vi "Norm VI Pt 2.vi"() -> ()   [LabVIEW 2026]
uses:
  <vilib>/DAQmx/read.llb/DAQmx Read (Digital 1D Bool 1Chan 1Samp).vi
  <vilib>/DAQmx/write.llb/DAQmx Write (Digital 1D Bool 1Chan 1Samp).vi
  <vilib>/numeric/Random Number (Range) U64.vi
  <vilib>/numeric/sub_Random U32.vi
  <vilib>/DAQmx/create/channels.llb/DAQmx Create Channel (DO-Digital Output).vi
  <vilib>/DAQmx/create/channels.llb/DAQmx Create Channel (DI-Digital Input).vi
  <vilib>/DAQmx/miscellaneous.llb/DAQmx Fill In Error Info.vi
panel:
  in  "stop":bool
  out "error out 5":errorcluster
  out "Numeric":i32
  out "Player 2":u64
  out "error out 4":errorcluster
  out "error out 3":errorcluster
  out "First Press?  2":bool
  out "Previous LED Position 2":u64
  out "Iteration Count 2":i32
  out "LEDs 2":bool[](array[boolean])
  out "HW Buttons  2":bool[](array[boolean])
  in  "?":bool
  in  "SW Buttons 2":bool[](array[boolean])
  out "Player 1":i8
  out "error out 2":errorcluster
  out "error out":errorcluster
  in  "SW Buttons":bool[](array[boolean])
  out "Debug Mode?":bool=TRUE
  out "First Press?":bool
  out "Previous LED Position":u64
  in  "Stop Program":bool
  out "HW Buttons":bool[](array[boolean])
  out "Iteration Count":i32
  out "LEDs":bool[](array[boolean])
  # "NI Speed of Light Demo"
  # "Press (Sticky Note) Button to Begin!"
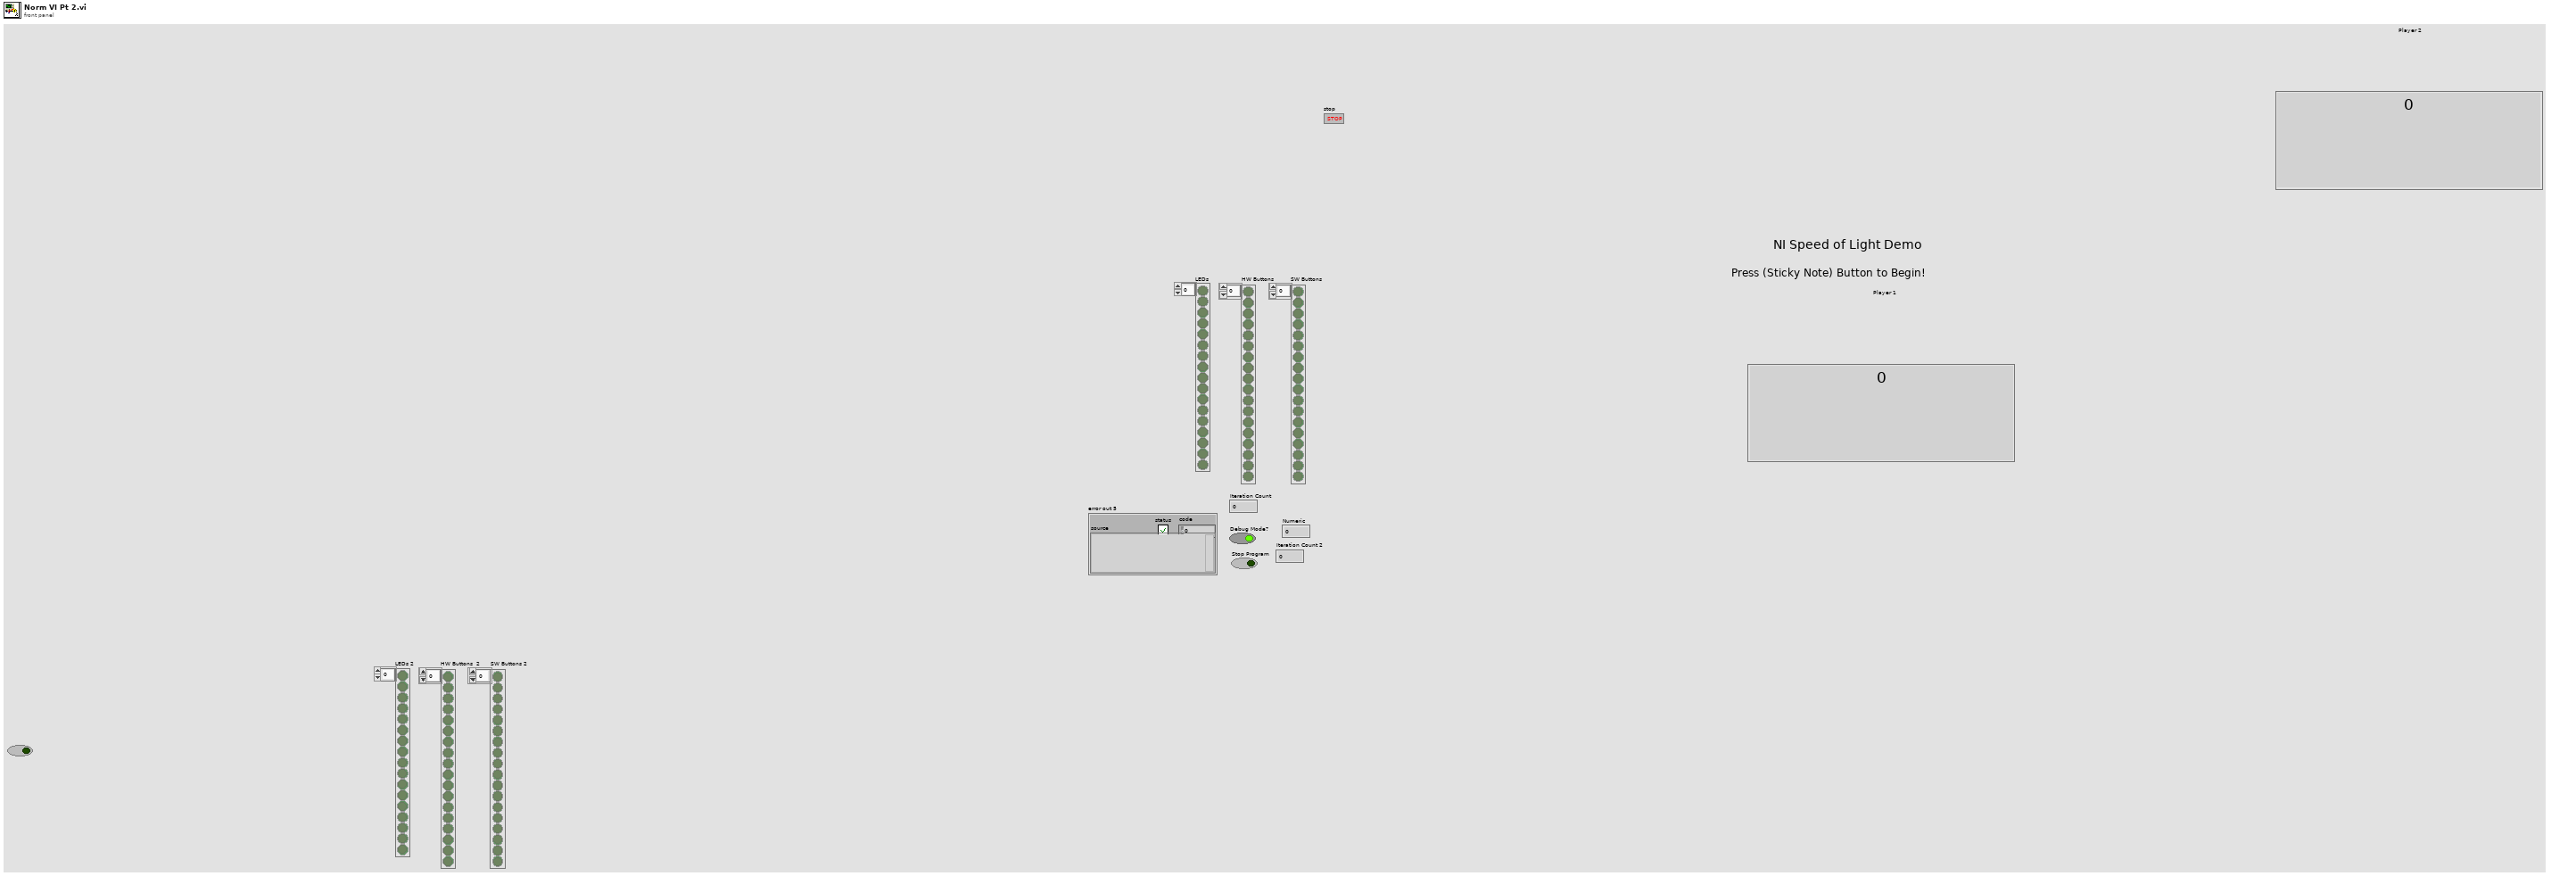
[diagram p1: front panel]
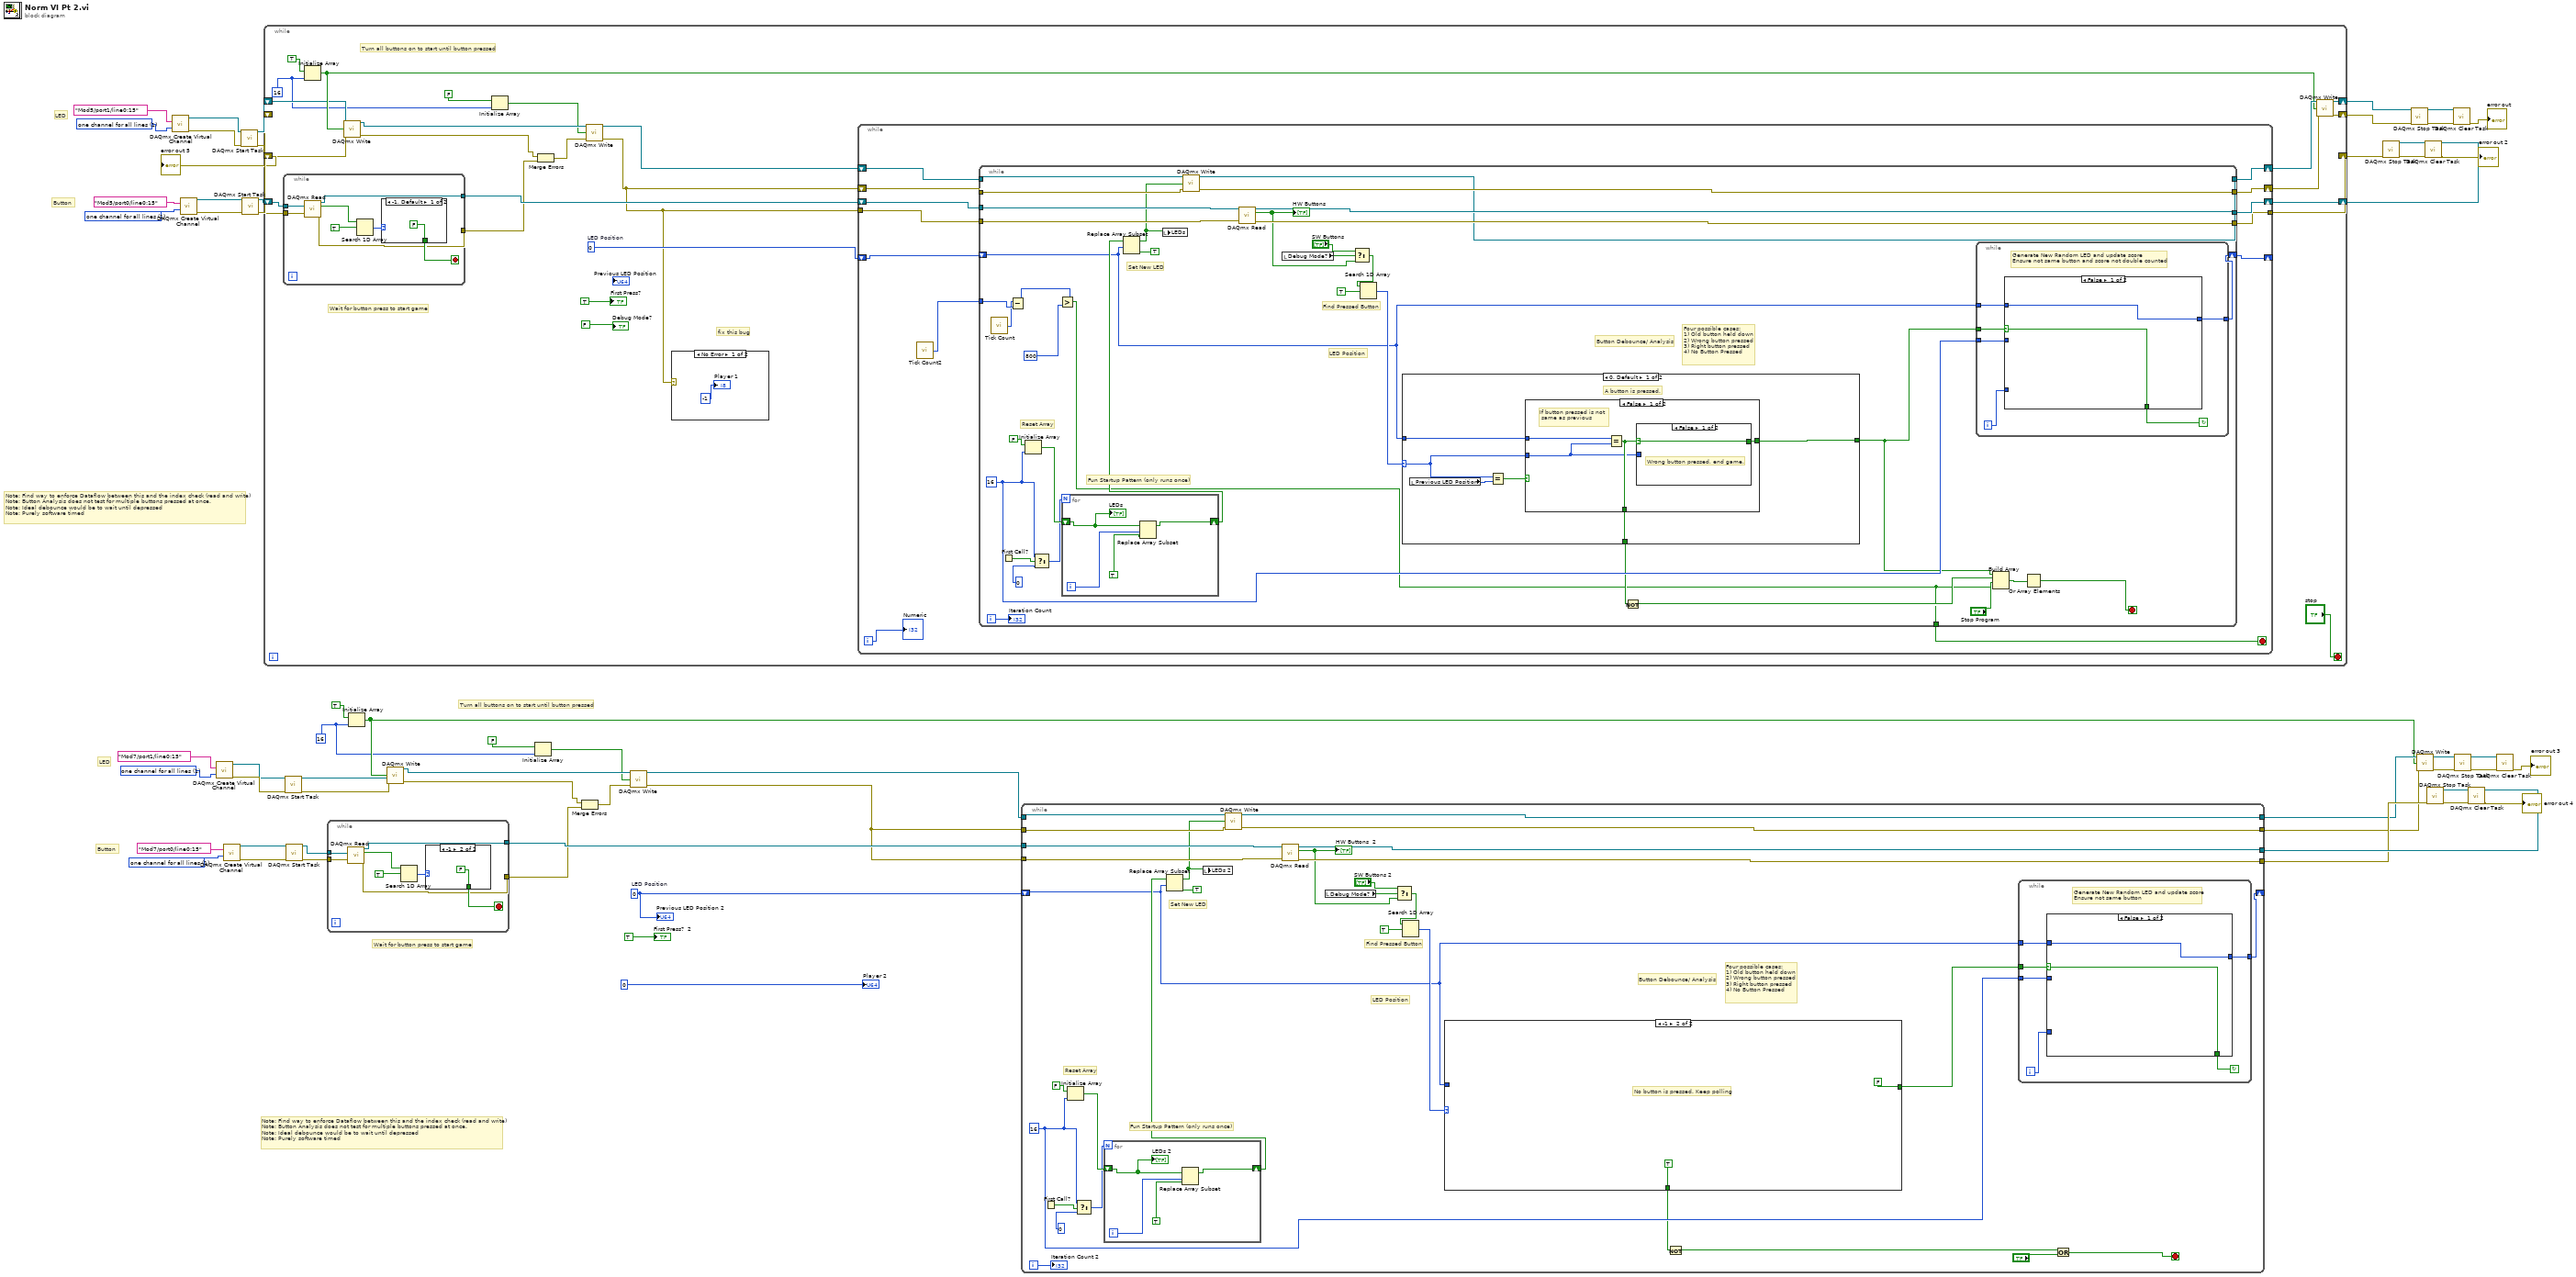
[diagram p0: block diagram]
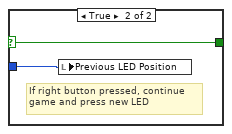
[diagram p3: hidden frame]
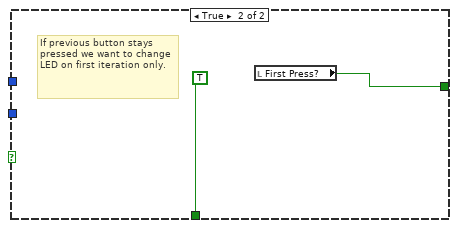
[diagram p4: hidden frame]
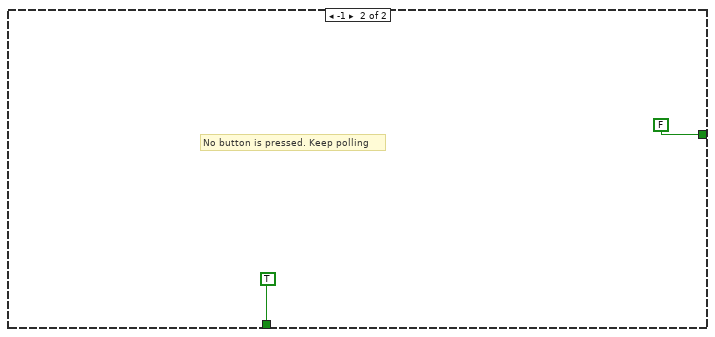
[diagram p5: hidden frame]
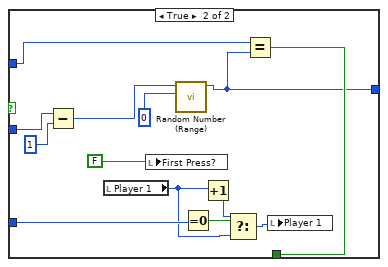
[diagram p6: hidden frame]
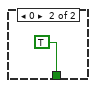
[diagram p7: hidden frame]
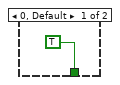
[diagram p8: hidden frame]
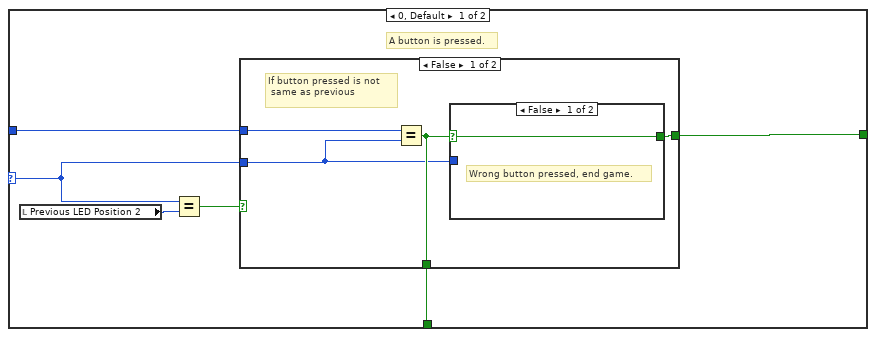
[diagram p9: hidden frame]
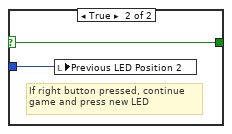
[diagram p10: hidden frame]
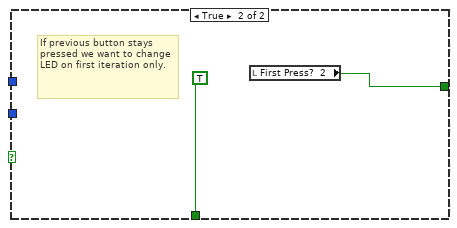
[diagram p11: hidden frame]
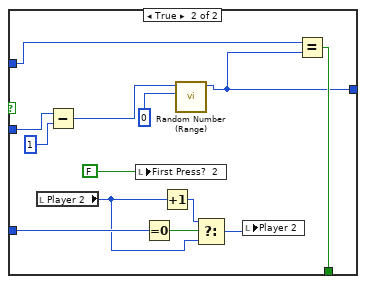
[diagram p12: hidden frame]
diagram:
  w6 = 16 ("dimension size")
  w28 = 1 items=["one channel for each line", "one channel for all lines"] ("line grouping")
  w29 = 1 items=["one channel for each line", "one channel for all lines"] ("line grouping")
  w27 = u64 0  # LED Position
  w50 = 1 items=["one channel for each line", "one channel for all lines"] ("line grouping")
  w51 = 1 items=["one channel for each line", "one channel for all lines"] ("line grouping")
  # "Turn all buttons on to start until button pressed"
  # "Wait for button press to start game"
  # "Note: Find way to enforce Dataflow between this and the index check (read and write)\nNote: Button Analysis does not test for multiple buttons pressed at once. \nNote: Ideal debounce would be to wait until depressed\nNote: Purely software timed"
  # "LED"
  # "Button"
  # "Note: Find way to enforce Dataflow between this and the index check (read and write)\nNote: Button Analysis does not test for multiple buttons pressed at once. \nNote: Ideal debounce would be to wait until depressed\nNote: Purely software timed"
  # "LED"
  # "Button"
  n1 = call-poly <vilib>:"DAQmx Create Virtual Channel.vi"("lines"=tag "Mod5/port1/line0:15", "line grouping"=w51) -> ("task out"=w3:refnum<k21>, "error out"=w2:errorcluster)  [unwired: 12 in]
  n2 = call-poly <vilib>:"DAQmx Create Virtual Channel.vi"("lines"=tag "Mod5/port0/line0:15", "line grouping"=w50) -> ("task out"=w60:refnum<k21>, "error out"=w61:errorcluster)  [unwired: 12 in]
  n3 = call-poly <vilib>:"DAQmx Create Virtual Channel.vi"("lines"=tag "Mod7/port1/line0:15", "line grouping"=w29) -> ("task out"=w35:refnum<k21>, "error out"=w36:errorcluster)  [unwired: 12 in]
  n4 = call-poly <vilib>:"DAQmx Create Virtual Channel.vi"("lines"=tag "Mod7/port0/line0:15", "line grouping"=w28) -> ("task out"=w41:refnum<k21>, "error out"=w42:errorcluster)  [unwired: 12 in]
  n5 = call <vilib>:"DAQmx Start Task.vi"("task/channels in"=w3, "error in"=w2) -> ("task out"=w45:refnum<k21>, "error out"=w1:errorcluster)  [unwired: 12 in]
  "error out 5" <- w1
  n6 = call <vilib>:"DAQmx Start Task.vi"("task/channels in"=w60, "error in"=w61) -> ("task out"=w43:refnum<k21>, "error out"=w44:errorcluster)  [unwired: 12 in]
  n7 = while {
    shift-right: [w82] -> w49
    shift-left: w45 -> [w77]
    shift-right: [w80] -> w48
    shift-left: w44 -> [w76]
    shift-right: [w87] -> w59
    shift-left: w43 -> [w75]
    shift-right: [w86] -> w56
    shift-left: w1 -> [w65]
    stop <- "stop" stop-if-true
    w68 = 16 ("dimension size")
    w64 = u64 0  # LED Position
    # "fix this bug"
    # "Turn all buttons on to start until button pressed"
    # "Wait for button press to start game"
    n8 = while {
      tunnel: w76 -> [w188]
      tunnel: w75 -> [w187]
      tunnel: [w182] -> w72
      tunnel: [w181] -> w74
      stop <- w183 stop-if-true
      n9 = call-poly <vilib>:"DAQmx Read.vi"("task/channels in"=w187, "error in"=w188) -> ("task out"=w181:refnum<k21>, "data"=w186:bool[], "error out"=w182:errorcluster)  [unwired: 11 in]
      n10 = Search 1D Array(1D array=w186, element=TRUE) -> (index of element=w184:i32)  [unwired: 1 in]
      n11 = case shown="-1, Default" w184 {
        tunnel: [FALSE TRUE] -> w183
        frame -1, Default {
        }
        frame 0 {
        }
      }
    }
    n12 = Initialize Array(TRUE, w68) -> (w78:bool[])
    n13 = call-poly <vilib>:"DAQmx Write.vi"("task/channels in"=w77, "data"=w78, "error in"=w65) -> ("task out"=w70:refnum<k21>, "error out"=w73:errorcluster)  [unwired: 10 in, 1 out]
    n14 = Initialize Array(FALSE ("element"), w68) -> (w66:bool[])
    n15 = Merge Errors(w73, w72) -> (w71:errorcluster)
    n16 = call-poly <vilib>:"DAQmx Write.vi"("task/channels in"=w70, "data"=w66, "error in"=w71) -> ("task out"=w69:refnum<k21>, "error out"=w62:errorcluster)  [unwired: 10 in, 1 out]
    n17 = case shown="No Error" w62 {
      frame No Error {
        "Player 1" <- i8 -1 ("Player 3")
      }
      frame Error {
      }
    }
    n18 = while {
      tunnel: [w100] -> w86
      shift-right: [w101] -> w87
      shift-left: w74 -> [w97]
      shift-right: [w98] -> w81
      shift-left: w62 -> [w96]
      shift-right: [w99] -> w85
      shift-left: w69 -> [w95]
      tunnel: w62 -> [w94]
      shift-right: [w91] -> _
      shift-left: w64 -> [w90]
      i -> [w93]
      stop <- w89 stop-if-true
      n19 = call "Tick Count2"() -> ("Tick Count(mSec)"=w92:u32)
      n20 = while {
        shift-right: [w136] -> w91
        shift-left: w90 -> [w118]
        tunnel: w94 -> [w135]
        tunnel: w97 -> [w134]
        tunnel: [w133] -> w101
        tunnel: [w132] -> w100
        tunnel: w96 -> [w131]
        tunnel: w95 -> [w130]
        tunnel: [w129] -> w98
        tunnel: [w128] -> w99
        tunnel: w92 -> [w104]
        tunnel: [w102] -> w89
        i -> [w138]
        stop <- w107 stop-if-true
        w122 = u64 16
        # "LED Position"
        # "Find Pressed Button"
        # "Four possible cases:\n1) Old button held down\n2) Wrong button pressed\n3) Right button pressed\n4) No Button Pressed"
        # "Fun Startup Pattern (only runs once)"
        # "Button Debounce/ Analysis"
        # "Set New LED"
        # "Reset Array"
        n21 = call "Tick Count"() -> ("Tick Count(mSec)"=w103:u32)
        n22 = First Call?() -> (First Call?: T/F=w125:bool)
        n23 = Subtract(x=w103, y=w104) -> (x-y=w106:u32)
        n24 = Initialize Array(FALSE, w122) -> (w126:bool[])
        n25 = Select(t=w122, s=w125, f=u64 0) -> (s? t:f=w123:u64)
        n26 = Greater?(x=w106, y=800) -> (0:w102:bool)
        n27 = for {
          N: w123 -> [_]
          shift-right: [w159] -> w121
          shift-left: w126 -> [w156]
          i -> [w158]
          n28 = Replace Array Subset(array=w156, new element=TRUE ("new element/subarray"), index=w158) -> (w159:bool[])
          "LEDs" <- w156
        }
        n29 = Replace Array Subset(array=w121, new element=TRUE ("new element/subarray"), index=w118) -> (w112:bool[])
        n30 = local write "LEDs"(w112) -> ()
        n31 = call-poly <vilib>:"DAQmx Write.vi"("task/channels in"=w130, "data"=w112, "error in"=w131) -> ("task out"=w128:refnum<k21>, "error out"=w129:errorcluster)  [unwired: 10 in, 1 out]
        n32 = call-poly <vilib>:"DAQmx Read.vi"("task/channels in"=w134, "error in"=w135) -> ("task out"=w133:refnum<k21>, "data"=w114:bool[], "error out"=w132:errorcluster)  [unwired: 11 in]
        "HW Buttons" <- w114
        n33 = local read "Debug Mode?"() -> (w116:bool)
        n34 = Select(t="SW Buttons", s=w116, f=w114) -> (s? t:f=w113:bool[])
        n35 = Search 1D Array(1D array=w113, element=TRUE) -> (index of element=w119:i32)  [unwired: 1 in]
        n36 = case shown="0, Default" w119 {
          selector: w119 -> [w140 _]
          tunnel: [w143 FALSE] -> w109
          tunnel: w118 -> [w141 _]
          tunnel: [w142 TRUE] -> w117
          frame 0, Default {
            # "A button is pressed."
            n37 = local read "Previous LED Position"() -> (w139:u64)
            n38 = Equal?(x=w140, y=w139) -> (x = y?=w144:bool)
            n39 = case shown="False" w144 {
              tunnel: [w145 w152] -> w143
              tunnel: [w147 TRUE] -> w142
              tunnel: w140 -> [w146 _]
              tunnel: w141 -> [w148 _]
              frame False {
                # "If button pressed is not\n same as previous"
                n40 = Equal?(x=w148, y=w146) -> (x = y?=w147:bool)
                n41 = case shown="False" w147 {
                  selector: w147 -> [w149 w150]
                  tunnel: w146 -> [_ w151]
                  tunnel: [w149 w150] -> w145
                  frame False {
                    # "Wrong button pressed, end game."
                  }
                  frame True {
                    # "If right button pressed, continue \ngame and press new LED"
                    n42 = local write "Previous LED Position"(w151) -> ()
                  }
                }
              }
              frame True {
                # "If previous button stays  pressed we want to change LED on first iteration only."
                n43 = local read "First Press?"() -> (w152:bool)
              }
            }
          }
          frame -1 {
            # "No button is pressed. Keep polling"
          }
        }
        n44 = Not(x=w117) -> (.not. x?=w111:bool)
        n45 = while {
          tunnel: w122 -> [w165]
          tunnel: [w164] -> w136
          tunnel: w118 -> [w163]
          tunnel: w109 -> [w161]
          i -> [w160]
          stop <- w162 continue-if-true
          # "Generate New Random LED and update score\nEnsure not same button and score not double counted"
          n46 = case shown="False" w161 {
            selector: w161 -> [w167 _]
            tunnel: w165 -> [_ w179]
            tunnel: [w166 w174] -> w164
            tunnel: w163 -> [w166 w176]
            tunnel: [w167 w175] -> w162
            tunnel: w160 -> [_ w169]
            frame False {
            }
            frame True {
              n47 = Subtract(x=w179, y=u64 1) -> (x-y=w177:u64)
              n48 = local read "Player 1"() -> (w168:i8)
              n49 = local write "First Press?"(FALSE ("First Press?  2")) -> ()
              n50 = call-poly <vilib>:"Random Number (Range).vi"("lower bound (0)"=u64 0, "upper bound (100)"=w177) -> ("number"=w174:u64)  [unwired: 9 in]
              n51 = Equal To 0?(x=w169) -> (x = 0?=w172:bool)
              n52 = Increment(x=w168) -> (x+1=w170:i8)
              n53 = Select(t=w170, s=w172, f=w168) -> (s? t:f=w171:i8)
              n54 = Equal?(x=w176, y=w174) -> (x = y?=w175:bool)
              n55 = local write "Player 1"(w171) -> ()
            }
          }
        }
        n56 = Build Array(w109, w111, "Stop Program", w102) -> (w108:bool[])
        n57 = Or Array Elements(Boolean array=w108) -> (logical OR=w107:bool)
        "Iteration Count" <- w138
      }
      "Numeric" <- w93
    }
    n58 = call-poly <vilib>:"DAQmx Write.vi"("task/channels in"=w85, "data"=w78, "error in"=w81) -> ("task out"=w82:refnum<k21>, "error out"=w80:errorcluster)  [unwired: 10 in, 1 out]
    "First Press?" <- TRUE ("First Press?  2")
    "Debug Mode?" <- FALSE ("Debug Mode? 2")
  }
  n59 = call <vilib>:"DAQmx Start Task.vi"("task/channels in"=w35, "error in"=w36) -> ("task out"=w17:refnum<k21>, "error out"=w16:errorcluster)  [unwired: 12 in]
  n60 = call <vilib>:"DAQmx Start Task.vi"("task/channels in"=w41, "error in"=w42) -> ("task out"=w14:refnum<k21>, "error out"=w15:errorcluster)  [unwired: 12 in]
  n61 = while {
    tunnel: w15 -> [w198]
    tunnel: w14 -> [w197]
    tunnel: [w192] -> w11
    tunnel: [w191] -> w13
    stop <- w193 stop-if-true
    n62 = call-poly <vilib>:"DAQmx Read.vi"("task/channels in"=w197, "error in"=w198) -> ("task out"=w191:refnum<k21>, "data"=w196:bool[], "error out"=w192:errorcluster)  [unwired: 11 in]
    n63 = Search 1D Array(1D array=w196, element=TRUE) -> (index of element=w194:i32)  [unwired: 1 in]
    n64 = case shown="-1" w194 {
      tunnel: [TRUE FALSE] -> w193
      frame 0, Default {
      }
      frame -1 {
      }
    }
  }
  n65 = Initialize Array(TRUE, w6) -> (w18:bool[])
  n66 = call-poly <vilib>:"DAQmx Write.vi"("task/channels in"=w17, "data"=w18, "error in"=w16) -> ("task out"=w8:refnum<k21>, "error out"=w12:errorcluster)  [unwired: 10 in, 1 out]
  n67 = Initialize Array(FALSE ("element"), w6) -> (w4:bool[])
  n68 = Merge Errors(w12, w11) -> (w10:errorcluster)
  n69 = call-poly <vilib>:"DAQmx Write.vi"("task/channels in"=w8, "data"=w4, "error in"=w10) -> ("task out"=w7:refnum<k21>, "error out"=w9:errorcluster)  [unwired: 10 in, 1 out]
  n70 = while {
    shift-right: [w229] -> _
    shift-left: w27 -> [w209]
    tunnel: w9 -> [w228]
    tunnel: w13 -> [w227]
    tunnel: [w226] -> w40
    tunnel: [w225] -> w37
    tunnel: w9 -> [w224]
    tunnel: w7 -> [w223]
    tunnel: [w222] -> w24
    tunnel: [w221] -> w32
    i -> [w231]
    stop <- w213 stop-if-true
    w215 = u64 16
    # "LED Position"
    # "Find Pressed Button"
    # "Four possible cases:\n1) Old button held down\n2) Wrong button pressed\n3) Right button pressed\n4) No Button Pressed"
    # "Fun Startup Pattern (only runs once)"
    # "Button Debounce/ Analysis"
    # "Set New LED"
    # "Reset Array"
    n71 = First Call?() -> (First Call?: T/F=w218:bool)
    n72 = Initialize Array(FALSE, w215) -> (w219:bool[])
    n73 = Select(t=w215, s=w218, f=u64 0) -> (s? t:f=w216:u64)
    n74 = for {
      N: w216 -> [_]
      shift-right: [w252] -> w214
      shift-left: w219 -> [w249]
      i -> [w251]
      n75 = Replace Array Subset(array=w249, new element=TRUE ("new element/subarray"), index=w251) -> (w252:bool[])
      "LEDs 2" <- w249
    }
    n76 = Replace Array Subset(array=w214, new element=TRUE ("new element/subarray"), index=w209) -> (w201:bool[])
    n77 = local write "LEDs 2"(w201) -> ()
    n78 = call-poly <vilib>:"DAQmx Write.vi"("task/channels in"=w223, "data"=w201, "error in"=w224) -> ("task out"=w221:refnum<k21>, "error out"=w222:errorcluster)  [unwired: 10 in, 1 out]
    n79 = call-poly <vilib>:"DAQmx Read.vi"("task/channels in"=w227, "error in"=w228) -> ("task out"=w226:refnum<k21>, "data"=w203:bool[], "error out"=w225:errorcluster)  [unwired: 11 in]
    "HW Buttons  2" <- w203
    n80 = local read "Debug Mode?"() -> (w205:bool)
    n81 = Select(t="SW Buttons 2", s=w205, f=w203) -> (s? t:f=w202:bool[])
    n82 = Search 1D Array(1D array=w202, element=TRUE) -> (index of element=w210:i32)  [unwired: 1 in]
    n83 = case shown="-1" w210 {
      selector: w210 -> [w233 _]
      tunnel: [w236 FALSE] -> w206
      tunnel: w209 -> [w234 _]
      tunnel: [w235 TRUE] -> w208
      frame 0, Default {
        # "A button is pressed."
        n84 = local read "Previous LED Position 2"() -> (w232:u64)
        n85 = Equal?(x=w233, y=w232) -> (x = y?=w237:bool)
        n86 = case shown="False" w237 {
          tunnel: [w238 w245] -> w236
          tunnel: [w240 TRUE] -> w235
          tunnel: w233 -> [w239 _]
          tunnel: w234 -> [w241 _]
          frame False {
            # "If button pressed is not\n same as previous"
            n87 = Equal?(x=w241, y=w239) -> (x = y?=w240:bool)
            n88 = case shown="False" w240 {
              selector: w240 -> [w242 w243]
              tunnel: w239 -> [_ w244]
              tunnel: [w242 w243] -> w238
              frame False {
                # "Wrong button pressed, end game."
              }
              frame True {
                # "If right button pressed, continue \ngame and press new LED"
                n89 = local write "Previous LED Position 2"(w244) -> ()
              }
            }
          }
          frame True {
            # "If previous button stays  pressed we want to change LED on first iteration only."
            n90 = local read "First Press?  2"() -> (w245:bool)
          }
        }
      }
      frame -1 {
        # "No button is pressed. Keep polling"
      }
    }
    n91 = Not(x=w208) -> (.not. x?=w207:bool)
    n92 = while {
      tunnel: w215 -> [w258]
      tunnel: [w257] -> w229
      tunnel: w209 -> [w256]
      tunnel: w206 -> [w254]
      i -> [w253]
      stop <- w255 continue-if-true
      # "Generate New Random LED and update score\nEnsure not same button"
      n93 = case shown="False" w254 {
        selector: w254 -> [w260 _]
        tunnel: w258 -> [_ w272]
        tunnel: [w259 w267] -> w257
        tunnel: w256 -> [w259 w269]
        tunnel: [w260 w268] -> w255
        tunnel: w253 -> [_ w265]
        frame False {
        }
        frame True {
          n94 = local read "Player 2"() -> (w261:u64)
          n95 = Subtract(x=w272, y=u64 1) -> (x-y=w270:u64)
          n96 = local write "First Press?  2"(FALSE ("First Press?  2")) -> ()
          n97 = Equal To 0?(x=w265) -> (x = 0?=w264:bool)
          n98 = Increment(x=w261) -> (x+1=w263:u64)
          n99 = call-poly <vilib>:"Random Number (Range).vi"("lower bound (0)"=u64 0, "upper bound (100)"=w270) -> ("number"=w267:u64)  [unwired: 9 in]
          n100 = Select(t=w263, s=w264, f=w261) -> (s? t:f=w262:u64)
          n101 = local write "Player 2"(w262) -> ()
          n102 = Equal?(x=w269, y=w267) -> (x = y?=w268:bool)
        }
      }
    }
    n103 = Or(x=w207, y="?") -> (x .or. y?=w213:bool)
    "Iteration Count 2" <- w231
  }
  n104 = call <vilib>:"DAQmx Stop Task.vi"("task/channels in"=w59, "error in"=w56) -> ("task out"=w58:refnum<k21>, "error out"=w57:errorcluster)  [unwired: 12 in]
  n105 = call <vilib>:"DAQmx Stop Task.vi"("task/channels in"=w49, "error in"=w48) -> ("task out"=w55:refnum<k21>, "error out"=w54:errorcluster)  [unwired: 12 in]
  n106 = call-poly <vilib>:"DAQmx Write.vi"("task/channels in"=w32, "data"=w18, "error in"=w24) -> ("task out"=w25:refnum<k21>, "error out"=w23:errorcluster)  [unwired: 10 in, 1 out]
  n107 = call <vilib>:"DAQmx Clear Task.vi"("task in"=w58, "error in"=w57) -> ("error out"=→"error out 2":errorcluster)  [unwired: 13 in]
  n108 = call <vilib>:"DAQmx Stop Task.vi"("task/channels in"=w40, "error in"=w37) -> ("task out"=w39:refnum<k21>, "error out"=w38:errorcluster)  [unwired: 12 in]
  n109 = call <vilib>:"DAQmx Clear Task.vi"("task in"=w55, "error in"=w54) -> ("error out"=→"error out":errorcluster)  [unwired: 13 in]
  n110 = call <vilib>:"DAQmx Stop Task.vi"("task/channels in"=w25, "error in"=w23) -> ("task out"=w34:refnum<k21>, "error out"=w33:errorcluster)  [unwired: 12 in]
  n111 = call <vilib>:"DAQmx Clear Task.vi"("task in"=w39, "error in"=w38) -> ("error out"=→"error out 4":errorcluster)  [unwired: 13 in]
  n112 = call <vilib>:"DAQmx Clear Task.vi"("task in"=w34, "error in"=w33) -> ("error out"=→"error out 3":errorcluster)  [unwired: 13 in]
  "Previous LED Position 2" <- w27
  "First Press?  2" <- TRUE ("First Press?  2")
  "Player 2" <- u64 0 ("Player 2 Score 2")
